vi "SwerveDrive2.0.vi"(6 "Right Trigger":dbl, 8 "RCW":dbl(slide) scale=-1.0..1.0, 9 "STR":dbl(slide) scale=-1.0..1.0, 10 "FWD":dbl(slide) scale=-1.0..1.0, 11 "Gyro":dbl) -> ()   [LabVIEW 2020]
uses:
  <vilib>/Rock Robotics/WPI/ThirdParty/ADI/ADIS16470/Typedef/ADIS16470 Data.ctl
  <vilib>/addons/control/pid/pid.llb/PID (DBL).vi
  <vilib>/addons/control/pid/NI_PID_pid.lvlib
panel:
  in  "Do X Pattern":bool
  out "Goal 4":dbl
  out "Goal 3":dbl
  out "Goal 2":dbl
  out "Goal 1":dbl
  in  "W4 PID":T1={"proportional gain (Kc)"=0.5, "integral time (Ti, min)"=0.0, "derivative time (Td, min)"=0.0}
  in  "W1 PID":T1={"proportional gain (Kc)"=0.5, "integral time (Ti, min)"=0.0, "derivative time (Td, min)"=0.0}
  in  "W2 PID":T1={"proportional gain (Kc)"=0.5, "integral time (Ti, min)"=0.0, "derivative time (Td, min)"=0.0}
  in  "W3 PID":T1={"proportional gain (Kc)"=0.5, "integral time (Ti, min)"=0.0, "derivative time (Td, min)"=0.0}
  out "ADIS16470 Value":T2
  out "W2 Encoder":dbl
  out "W1 Encoder":dbl
  out "WA 4":dbl
  out "WA 3":dbl
  out "WA 2":dbl
  out "WA 1":dbl
  out "WS 4":dbl
  out "WS 3":dbl
  out "WS 2":dbl
  out "WS 1":dbl
  out "W4 Encoder":dbl
  out "W3 Encoder":dbl
  # "0.5\n0\n0\nfor all"
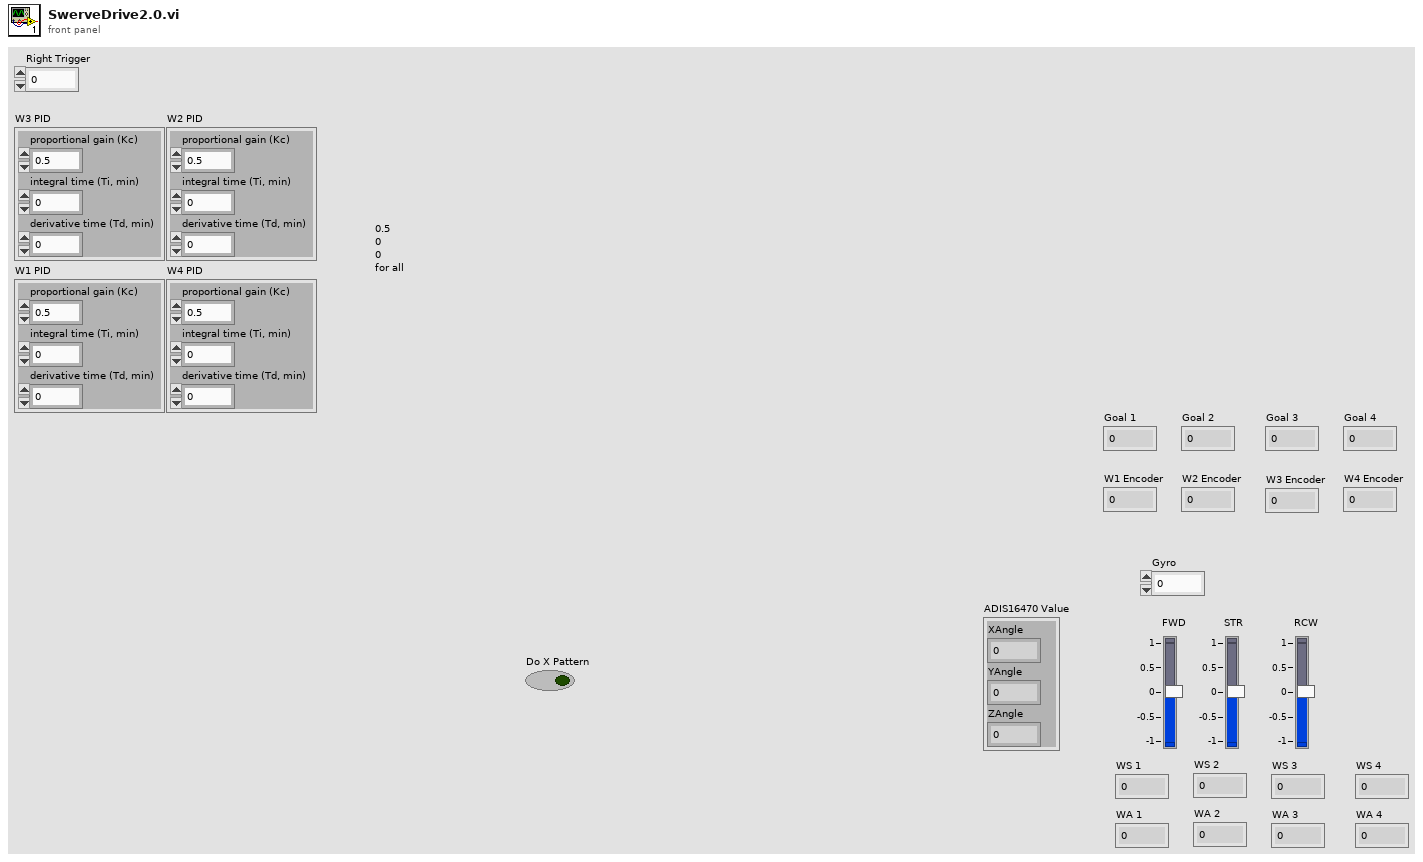
[diagram p1: front panel]
types:
  T1 = cluster{"proportional gain (Kc)":dbl, "integral time (Ti, min)":dbl, "derivative time (Td, min)":dbl}
  T2 = typedef "ADIS16470 Data.ctl" = cluster{"XAngle":dbl, "YAngle":dbl, "ZAngle":dbl}
  T3 = typedef "WPI_JoystickDevRef.ctl" = cluster{"Device":T4}
  T4 = typedef "WPI_JoystickDeviceEnum.ctl" = enum16{"USB 0", "USB 1", "USB 2", "USB 3", "USB 4", "USB 5"}
  T5 = typedef "ADIS16470 Device Reference.ctl" = cluster{"DevStatus":errorcluster, "Hardware Config":T6, "Calibration Complete":refnum<notifier>, "Status Reference":refnum<data-value>, "Data Reference":refnum<data-value>, "Sychronous Process VI":T10, "Cmd FIFO":refnum<k33>, "Source":T11, "Data FIFO":refnum<k33>, "Calibration Time (ms)":u32, "Data Reference":refnum<data-value>}
  T6 = typedef "ADIS16470 Hardware Configuration.ctl" = cluster{"SPI Clock Rate (Hz)":dbl, "IMU SPI Mode (3)":T7, "IMU Reset Pin":T8, "IMU SPI Bus":T9, "IMU Data Ready Pin":T8, "Stall Config":cluster{"Pow2BytesPerRead":u8, "StallTicks":u16, "CsToSclkTicks":u8}}
  T7 = typedef "WPI_SPIMode.ctl" = enum16{"Mode 0 (Clk Idle Low,Sample on Leading)", "Mode 1 (Clk Idle Low,Sample on Trailing)", "Mode 2 (Clk Idle High,Sample on Leading)", "Mode 3 (Clk Idle High,Sample on Trailing)"}
  T8 = typedef "FPGA_DIOChannel.ctl" = enum8{"DIO 0", "DIO 1", "DIO 2", "DIO 3", "DIO 4", "DIO 5", "DIO 6", "DIO 7", "DIO 8", "DIO 9", "DIO MXP 0", "DIO MXP 1", "DIO MXP 2", "DIO MXP 3", "DIO MXP 4", "DIO MXP 5", "DIO MXP 6", "DIO MXP 7", "DIO MXP 8", "DIO MXP 9", "DIO MXP 10", "DIO MXP 11", "DIO MXP 12", "DIO MXP 13", "DIO MXP 14", "DIO MXP 15", "SPI Port CS1", "SPI Port CS2", "SPI Port CS3", "SPI Port MISO", "SPI Port MOSI", "Invalid"}
  T9 = typedef "spi_bus.ctl" = enum16{"SPI On-Board, CS0", "SPI On-Board, CS1", "SPI On-Board, CS2", "SPI On-Board, CS3", "SPI MXP", "Invalid"}
  T10 = typedef "ADIS16470 Process.ctl" = refnum<vi>
  T11 = typedef "FPGA_CounterEncoderSourceConvertionLVSourceType.ctl" = cluster{"DevStatus":errorcluster, "AnalogTriggerMode?":bool, "DigitalMode":cluster{"DIO Channel":T12}, "AnalogTriggerMode":cluster{"AnalogTriggerIndex":T13, "OutputType":T14}}
  T12 = typedef "FPGA_DIODigitalSourceChannel.ctl" = enum8{"DIO 0", "DIO 1", "DIO 2", "DIO 3", "DIO 4", "DIO 5", "DIO 6", "DIO 7", "DIO 8", "DIO 9", "DIO MXP 0", "DIO MXP 1", "DIO MXP 2", "DIO MXP 3", "DIO MXP 4", "DIO MXP 5", "DIO MXP 6", "DIO MXP 7", "DIO MXP 8", "DIO MXP 9", "DIO MXP 10", "DIO MXP 11", "DIO MXP 12", "DIO MXP 13", "DIO MXP 14", "DIO MXP 15", "SPI Port CS1", "SPI Port CS2", "SPI Port CS3", "SPI Port MISO", "SPI Port MOSI", "Disabled"}
  T13 = typedef "FPGA_AnalogTriggerIndex.ctl" = enum8{"Trig 0", "Trig 1", "Trig 2", "Trig 3", "Trig 4", "Trig 5", "Trig 6", "Trig 7", "Invalid"}
  T14 = typedef "FPGA_AnalogTriggerOutType.ctl" = enum16{"InWindow", "TriggerState", "Rising", "Falling"}
  T15 = typedef "WPI_MotorControlDeviceRef.ctl" = cluster{"DeviceStatus":errorcluster, "Type":T16, "PWM":cluster{"PWM Channel":T17, "DeadBand":T18}, "CAN":cluster{"Device Number":u8, "SetOutput VI Ref":variant, "GetOutput VI Ref":variant, "Enable VI Ref":variant, "Disable VI Ref":variant, "Data":variant}, "Invert":bool, "DIO PWM":cluster{"PWM \"Enable\" Channel":T17, "DIOChannel":T8, "PWM Rate":dbl}}
  T16 = typedef "WPI_MotorControlType.ctl" = enum16{"PWM", "CAN", "DIO PWM"}
  T17 = typedef "FPGA_DIOPWMChannel.ctl" = enum8{"PWM 0", "PWM 1", "PWM 2", "PWM 3", "PWM 4", "PWM 5", "PWM 6", "PWM 7", "PWM 8", "PWM 9", "PWM MXP 0", "PWM MXP 1", "PWM MXP 2", "PWM MXP 3", "PWM MXP 4", "PWM MXP 5", "PWM MXP 6", "PWM MXP 7", "PWM MXP 8", "PWM MXP 9", "Invalid"}
  T18 = typedef "WPI_PWMDeadband.ctl" = cluster{"Name":string, "maxPositivePwm":i32, "minPositivePwm":i32, "centerPwm":i32, "maxNegativePwm":i32, "minNegativePwm":i32, "angularRange":u16}
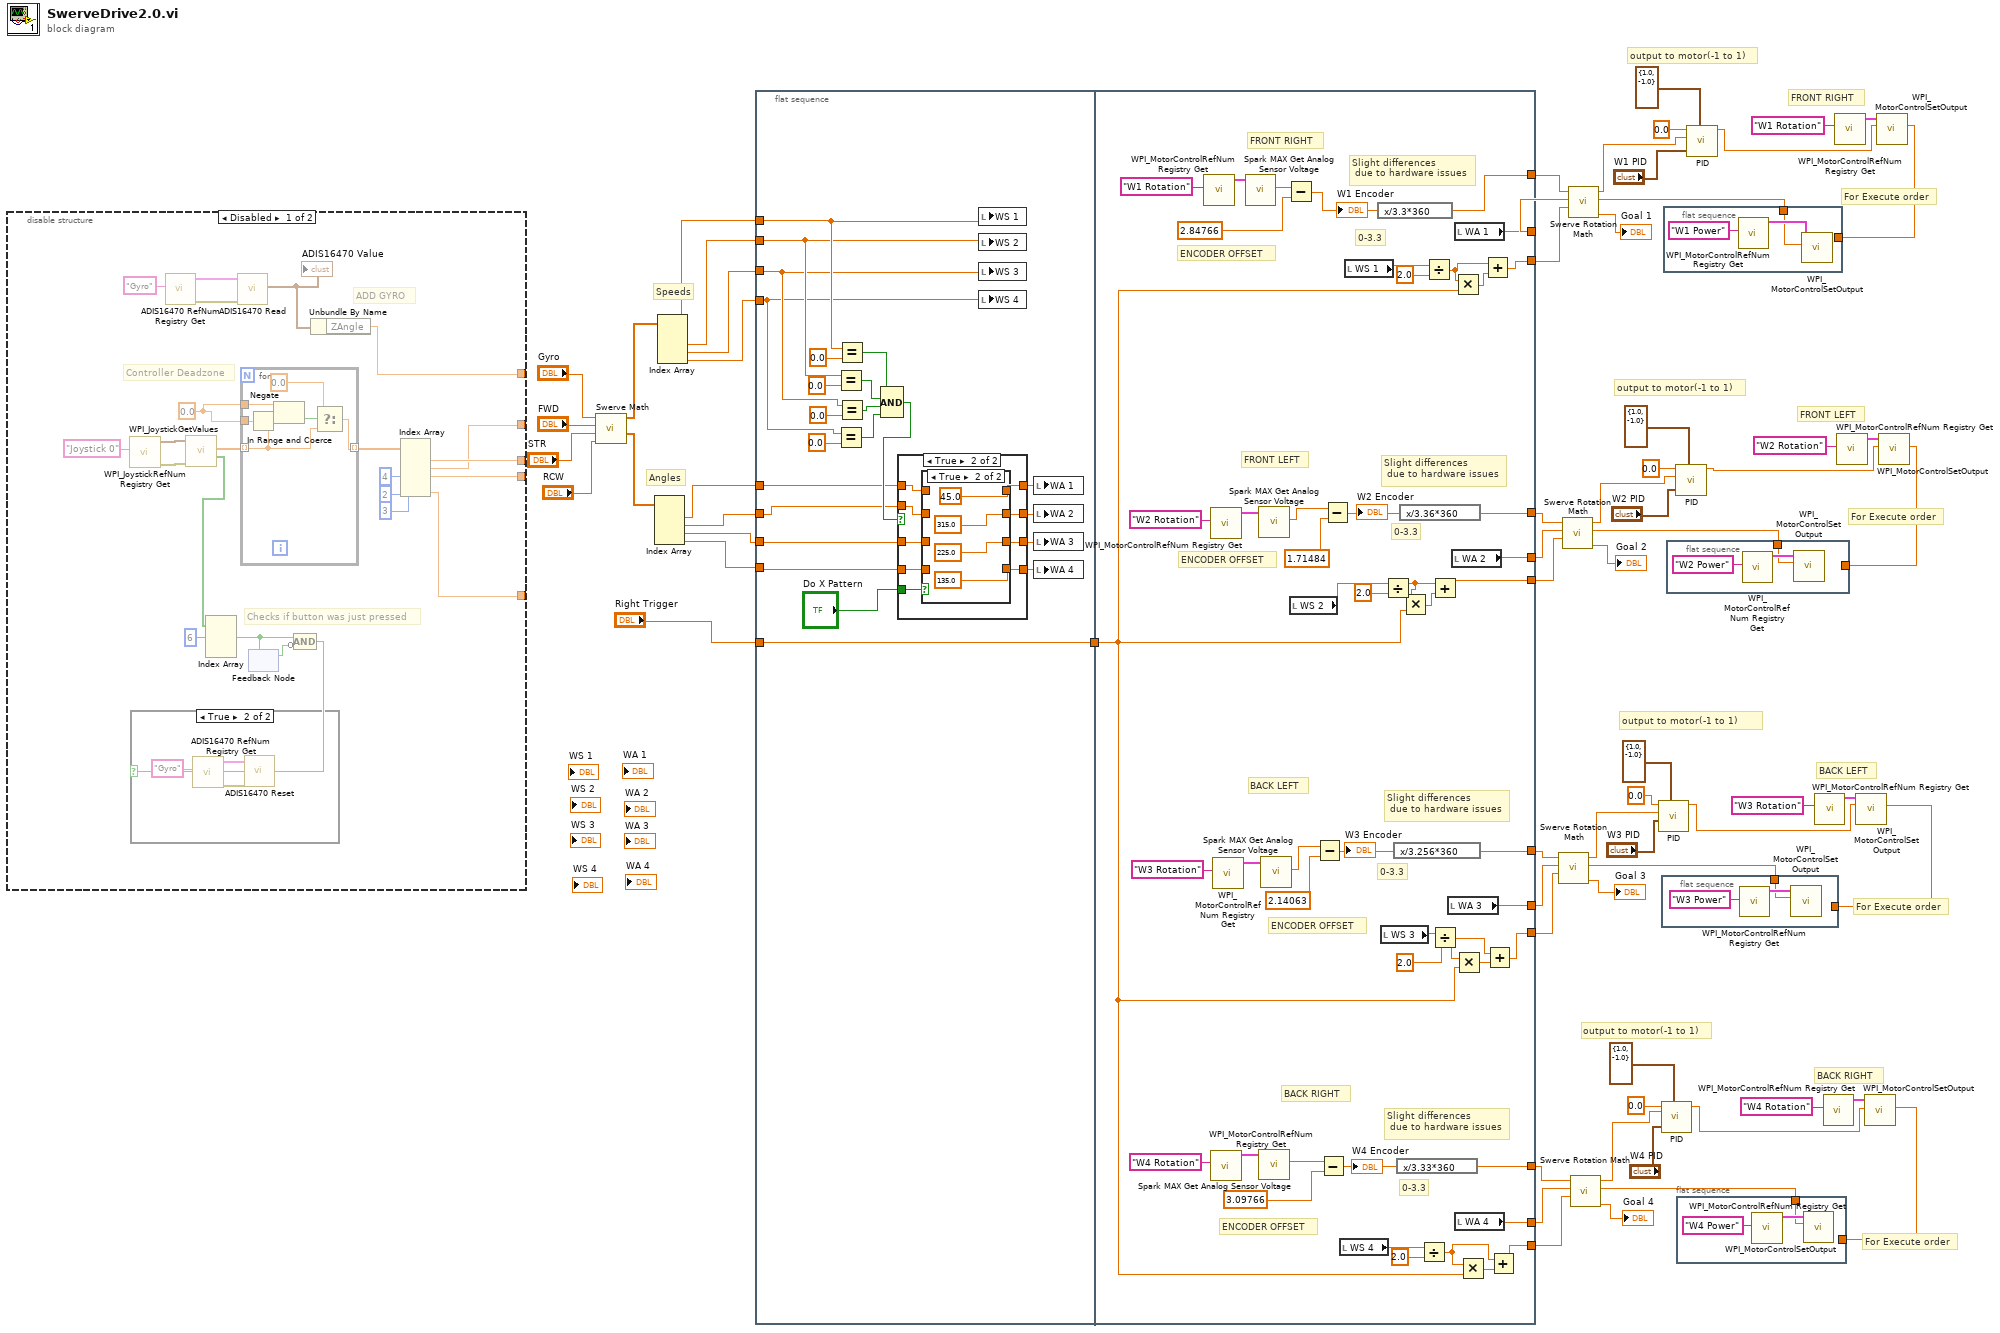
[diagram p0: block diagram]
diagram:
  # "output to motor(-1 to 1)"
  # "BACK RIGHT"
  # "BACK LEFT"
  # "FRONT LEFT"
  # "FRONT RIGHT"
  # "output to motor(-1 to 1)"
  # "output to motor(-1 to 1)"
  # "output to motor(-1 to 1)"
  # "For Execute order"
  # "For Execute order"
  # "For Execute order"
  # "For Execute order"
  # "Angles"
  # "Speeds"
  n1 = disable-structure shown="Disabled" {
    disable-tunnel: [w88 _] -> _
    disable-tunnel: [w87 _] -> _
    disable-tunnel: [w86 _] -> _
    disable-tunnel: [w75 _] -> _
    disable-tunnel: [w72 _] -> _
    frame Disabled {
      w81 = 0.0 ("upper limit")
      # "Checks if button was just pressed"
      # "Controller Deadzone"
      # "ADD GYRO"
      n2 = call <vilib>:"WPI_JoystickRefNum Registry Get.vi"("refnum name"="Joystick 0") -> ("error out"=w91:errorcluster, "JoystickDevRef"=w90:T3)  [unwired: 9 in]
      n3 = call <vilib>:"ADIS16470 RefNum Registry Get.vi"("refnum name"="Gyro") -> ("error out"=w71:errorcluster, "ADIS16470DevRef out"=w69:T5)  [unwired: 9 in]
      n4 = call <vilib>:"WPI_JoystickGetValues.vi"("error in (no error)"=w91, "JoystickDevRef"=w90) -> ("Buttons"=w80:bool[], "Axes"=w83:dbl[])  [unwired: 5 in, 3 out]
      n5 = Index Array(array=w80, index #1=6 ("index")) -> (element #1=w78:bool)  [unwired: 2 in, 2 out]
      n6 = call <vilib>:"ADIS16470 Read.vi"("error in (no error)"=w71, "ADIS16470DevRef"=w69) -> ("ADIS16470 Value"=w84:T2)  [unwired: 6 in, 3 out]
      "ADIS16470 Value" <- w84
      n7 = for {
        tunnel: w83 -> [w96] mode=indexing
        tunnel: [w95] -> w82 mode=indexing
        tunnel: w81 -> [w101]
        tunnel: w81 -> [w100]
        n8 = Negate(x=w100) -> (-x=w99:dbl)
        n9 = In Range and Coerce(upper limit=w101, x=w96, lower limit=w99) -> (In Range?=w98:bool)  [unwired: 1 out]
        n10 = Select(t=0.0, s=w98, f=w96) -> (s? t:f=w95:dbl)
      }
      n11 = feedback #1() -> (w77:bool)  [unwired: 1 in]
      n12 = feedback-in #1(w78) -> ()
      n13 = Compound Arithmetic op=AND(w78, invert w77) -> (w76:bool)
      n14 = case shown="True" w76 {
        frame False {
        }
        frame True {
          n15 = call <vilib>:"ADIS16470 RefNum Registry Get.vi"("refnum name"="Gyro") -> ("error out"=w93:errorcluster, "ADIS16470DevRef out"=w92:T5)  [unwired: 9 in]
          n16 = call <vilib>:"ADIS16470 Reset.vi"("error in (no error)"=w93, "ADIS16470DevRef"=w92) -> ()  [unwired: 8 in, 2 out]
        }
      }
      n17 = Unbundle By Name(w84) -> ("ZAngle"=w75:dbl)
      n18 = Index Array(array=w82, index #3=4 ("index"), index #4=2 ("index"), index #5=3 ("index")) -> (element #1=w88:dbl, element #2=w86:dbl, element #3=w87:dbl, element #5=w72:dbl)  [unwired: 2 in, 1 out]
    }
    frame Enabled {
    }
  }
  n19 = call "Swerve Math.vi"("Gyro"="Gyro", "FWD"="FWD", "STR"="STR", "RCW"="RCW") -> ("Wheel Speeds"=w68:dbl[], "Wheel Angles"=w67:dbl[])  [unwired: 5 in]
  n20 = Index Array(array=w67) -> (element #1=w51:dbl, element #2=w52:dbl, element #3=w53:dbl, element #4=w54:dbl)  [unwired: 4 in]
  n21 = Index Array(array=w68) -> (element #1=w49:dbl, element #2=w3:dbl, element #3=w4:dbl, element #4=w50:dbl)  [unwired: 4 in]
  n22 = flat-sequence {
    tunnel: w54 -> [w103]
    tunnel: w53 -> [w106]
    tunnel: w52 -> [w108]
    tunnel: w51 -> [w110]
    tunnel: w50 -> [w112]
    tunnel: w4 -> [w113]
    tunnel: w49 -> [w115]
    tunnel: w3 -> [w114]
    tunnel: "Right Trigger" -> [w124]
    tunnel: [w124] -> w2
    tunnel: [w194] -> w47
    tunnel: [w193] -> w41
    tunnel: [w192] -> w35
    tunnel: [w191] -> w30
    tunnel: [w190] -> w36
    tunnel: [w189] -> w28
    tunnel: [w172] -> w42
    tunnel: [w171] -> w48
    tunnel: [w154] -> w46
    tunnel: [w158] -> w40
    tunnel: [w150] -> w34
    tunnel: [w148] -> w29
    tunnel: w2 -> [w146]
    frame #0 {
      n23 = Equal?(x=w114, y=0.0) -> (x = y?=w120:bool)
      n24 = Equal?(x=w112, y=0.0) -> (x = y?=w116:bool)
      n25 = Equal?(x=w115, y=0.0) -> (x = y?=w123:bool)
      n26 = Equal?(x=w113, y=0.0) -> (x = y?=w117:bool)
      n27 = Compound Arithmetic op=AND(w123, w120, w117, w116) -> (w111:bool)
      n28 = case shown="True" w111 {
        tunnel: w110 -> [w128 w132]
        tunnel: [w128 w137] -> w109
        tunnel: w108 -> [w127 w131]
        tunnel: [w127 w136] -> w107
        tunnel: w106 -> [w126 w130]
        tunnel: [w126 w135] -> w105
        tunnel: w103 -> [w125 w129]
        tunnel: [w125 w134] -> w104
        tunnel: "Do X Pattern" -> [_ w133]
        frame False {
        }
        frame True {
          n29 = case shown="True" w133 {
            tunnel: [w141 45.0] -> w137
            tunnel: [w140 315.0] -> w136
            tunnel: [w139 225.0] -> w135
            tunnel: [w138 135.0] -> w134
            tunnel: w132 -> [w141 _]
            tunnel: w131 -> [w140 _]
            tunnel: w130 -> [w139 _]
            tunnel: w129 -> [w138 _]
            frame False {
            }
            frame True {
            }
          }
        }
      }
      n30 = local write "WS 1"(w115) -> ()
      n31 = local write "WS 2"(w114) -> ()
      n32 = local write "WS 3"(w113) -> ()
      n33 = local write "WS 4"(w112) -> ()
      n34 = local write "WA 1"(w109) -> ()
      n35 = local write "WA 2"(w107) -> ()
      n36 = local write "WA 3"(w105) -> ()
      n37 = local write "WA 4"(w104) -> ()
    }
    frame #1 {
      # "Slight differences\n due to hardware issues"
      # "Slight differences\n due to hardware issues"
      # "Slight differences\n due to hardware issues"
      # "Slight differences\n due to hardware issues"
      # "BACK RIGHT"
      # "BACK LEFT"
      # "FRONT LEFT"
      # "FRONT RIGHT"
      # "ENCODER OFFSET"
      # "ENCODER OFFSET"
      # "ENCODER OFFSET"
      # "ENCODER OFFSET"
      # "0-3.3"
      # "0-3.3"
      # "0-3.3"
      # "0-3.3"
      n38 = call <vilib>:"WPI_MotorControlRefNum Registry Get.vi"("refnum name"="W1 Rotation") -> ("MotorControlDevRef"=w188:T15)  [unwired: 9 in, 1 out]
      n39 = call <vilib>:"WPI_MotorControlRefNum Registry Get.vi"("refnum name"="W2 Rotation") -> ("MotorControlDevRef"=w173:T15)  [unwired: 9 in, 1 out]
      n40 = call <vilib>:"WPI_MotorControlRefNum Registry Get.vi"("refnum name"="W4 Rotation") -> ("MotorControlDevRef"=w183:T15)  [unwired: 9 in, 1 out]
      n41 = call <vilib>:"WPI_MotorControlRefNum Registry Get.vi"("refnum name"="W3 Rotation") -> ("MotorControlDevRef"=w185:T15)  [unwired: 9 in, 1 out]
      n42 = call <vilib>:"Spark MAX Get Analog Sensor Voltage.vi"("MotorControlDevRef in"=w188) -> ("Analog Sensor Voltage"=w180:dbl)  [unwired: 7 in, 3 out]
      n43 = call <vilib>:"Spark MAX Get Analog Sensor Voltage.vi"("MotorControlDevRef in"=w173) -> ("Analog Sensor Voltage"=w178:dbl)  [unwired: 7 in, 3 out]
      n44 = call <vilib>:"Spark MAX Get Analog Sensor Voltage.vi"("MotorControlDevRef in"=w183) -> ("Analog Sensor Voltage"=w179:dbl)  [unwired: 7 in, 3 out]
      n45 = call <vilib>:"Spark MAX Get Analog Sensor Voltage.vi"("MotorControlDevRef in"=w185) -> ("Analog Sensor Voltage"=w181:dbl)  [unwired: 7 in, 3 out]
      n46 = Subtract(x=w180, y=2.84766) -> (x-y=w166:dbl)
      "W1 Encoder" <- w166
      n47 = local read "WS 2"() -> (w176:dbl)
      n48 = Subtract(x=w181, y=2.14063) -> (x-y=w164:dbl)
      "W3 Encoder" <- w164
      n49 = Subtract(x=w179, y=3.09766 ("x")) -> (x-y=w163:dbl)
      "W4 Encoder" <- w163
      n50 = Subtract(x=w178, y=1.71484) -> (x-y=w165:dbl)
      "W2 Encoder" <- w165
      n51 = local read "WS 4"() -> (w174:dbl)
      n52 = local read "WS 1"() -> (w177:dbl)
      n53 = expression code="x/3.3*360"(w166) -> (w171:dbl)
      n54 = local read "WS 3"() -> (w175:dbl)
      n55 = Divide(x=w176, y=2.0) -> (x/y=w156:dbl)
      n56 = expression code="x/3.256*360"(w164) -> (w190:dbl)
      n57 = expression code="x/3.33*360"(w163) -> (w189:dbl)
      n58 = expression code="x/3.36*360"(w165) -> (w172:dbl)
      n59 = Multiply(x=w156, y=w146) -> (x*y=w157:dbl)
      n60 = Divide(x=w174, y=2.0) -> (x/y=w147:dbl)
      n61 = Divide(x=w177, y=2.0) -> (x/y=w153:dbl)
      n62 = Add(x=w156, y=w157) -> (x+y=w158:dbl)
      n63 = Divide(x=w175, y=2.0) -> (x/y=w151:dbl)
      n64 = local read "WA 3"() -> (w192:dbl)
      n65 = local read "WA 2"() -> (w193:dbl)
      n66 = Multiply(x=w153, y=w146) -> (x*y=w155:dbl)
      n67 = Multiply(x=w151, y=w146) -> (x*y=w152:dbl)
      n68 = local read "WA 1"() -> (w194:dbl)
      n69 = local read "WA 4"() -> (w191:dbl)
      n70 = Multiply(x=w147, y=w146) -> (x*y=w149:dbl)
      n71 = Add(x=w153, y=w155) -> (x+y=w154:dbl)
      n72 = Add(x=w151, y=w152) -> (x+y=w150:dbl)
      n73 = Add(x=w147, y=w149) -> (x+y=w148:dbl)
    }
  }
  n74 = call "Swerve Rotation Math.vi"("Wheel Speed"=w34, "Wheel Angle"=w35, "Encoder"=w36) -> ("Goal"=→"Goal 3":dbl, "Wheel Speed"=w32:dbl, "Difference"=w33:dbl)  [unwired: 6 in]
  n75 = call "Swerve Rotation Math.vi"("Wheel Speed"=w40, "Wheel Angle"=w41, "Encoder"=w42) -> ("Goal"=→"Goal 2":dbl, "Wheel Speed"=w38:dbl, "Difference"=w39:dbl)  [unwired: 6 in]
  n76 = call "Swerve Rotation Math.vi"("Wheel Speed"=w46, "Wheel Angle"=w47, "Encoder"=w48) -> ("Goal"=→"Goal 1":dbl, "Wheel Speed"=w44:dbl, "Difference"=w43:dbl)  [unwired: 6 in]
  n77 = call "Swerve Rotation Math.vi"("Wheel Speed"=w29, "Wheel Angle"=w30, "Encoder"=w28) -> ("Goal"=→"Goal 4":dbl, "Wheel Speed"=w9:dbl, "Difference"=w26:dbl)  [unwired: 6 in]
  n78 = call-poly <vilib>:"PID.vi"("output range"=cluster{"output high":dbl, "output low":dbl} {"output high"=1.0, "output low"=-1.0}, "PID gains"="W3 PID", "process variable"=w33, "setpoint"=0.0) -> ("output"=w16:dbl)  [unwired: 6 in, 1 out]
  n79 = flat-sequence {
    tunnel: w14 -> [_]
    tunnel: w32 -> [w195]
    frame #0 {
      n80 = call <vilib>:"WPI_MotorControlRefNum Registry Get.vi"("refnum name"="W3 Power") -> ("MotorControlDevRef"=w196:T15)  [unwired: 9 in, 1 out]
      n81 = call <vilib>:"WPI_MotorControlSetOutput.vi"("Output"=w195, "MotorControlDevRef"=w196) -> ()  [unwired: 7 in, 3 out]
    }
  }
  n82 = call-poly <vilib>:"PID.vi"("output range"=cluster{"output high":dbl, "output low":dbl} {"output high"=1.0, "output low"=-1.0}, "PID gains"="W4 PID", "process variable"=w26, "setpoint"=0.0) -> ("output"=w12:dbl)  [unwired: 6 in, 1 out]
  n83 = flat-sequence {
    tunnel: w22 -> [_]
    tunnel: w44 -> [w198]
    frame #0 {
      n84 = call <vilib>:"WPI_MotorControlRefNum Registry Get.vi"("refnum name"="W1 Power") -> ("MotorControlDevRef"=w199:T15)  [unwired: 9 in, 1 out]
      n85 = call <vilib>:"WPI_MotorControlSetOutput.vi"("Output"=w198, "MotorControlDevRef"=w199) -> ()  [unwired: 7 in, 3 out]
    }
  }
  n86 = flat-sequence {
    tunnel: w18 -> [_]
    tunnel: w38 -> [w201]
    frame #0 {
      n87 = call <vilib>:"WPI_MotorControlRefNum Registry Get.vi"("refnum name"="W2 Power") -> ("MotorControlDevRef"=w202:T15)  [unwired: 9 in, 1 out]
      n88 = call <vilib>:"WPI_MotorControlSetOutput.vi"("Output"=w201, "MotorControlDevRef"=w202) -> ()  [unwired: 7 in, 3 out]
    }
  }
  n89 = call-poly <vilib>:"PID.vi"("output range"=cluster{"output high":dbl, "output low":dbl} {"output high"=1.0, "output low"=-1.0}, "PID gains"="W2 PID", "process variable"=w39, "setpoint"=0.0) -> ("output"=w20:dbl)  [unwired: 6 in, 1 out]
  n90 = flat-sequence {
    tunnel: w10 -> [_]
    tunnel: w9 -> [w204]
    frame #0 {
      n91 = call <vilib>:"WPI_MotorControlRefNum Registry Get.vi"("refnum name"="W4 Power") -> ("MotorControlDevRef"=w205:T15)  [unwired: 9 in, 1 out]
      n92 = call <vilib>:"WPI_MotorControlSetOutput.vi"("Output"=w204, "MotorControlDevRef"=w205) -> ()  [unwired: 7 in, 3 out]
    }
  }
  n93 = call-poly <vilib>:"PID.vi"("output range"=cluster{"output high":dbl, "output low":dbl} {"output high"=1.0, "output low"=-1.0}, "PID gains"="W1 PID", "process variable"=w43, "setpoint"=0.0) -> ("output"=w24:dbl)  [unwired: 6 in, 1 out]
  n94 = call <vilib>:"WPI_MotorControlRefNum Registry Get.vi"("refnum name"="W3 Rotation") -> ("MotorControlDevRef"=w17:T15)  [unwired: 9 in, 1 out]
  n95 = call <vilib>:"WPI_MotorControlRefNum Registry Get.vi"("refnum name"="W4 Rotation") -> ("MotorControlDevRef"=w13:T15)  [unwired: 9 in, 1 out]
  n96 = call <vilib>:"WPI_MotorControlRefNum Registry Get.vi"("refnum name"="W1 Rotation") -> ("MotorControlDevRef"=w25:T15)  [unwired: 9 in, 1 out]
  n97 = call <vilib>:"WPI_MotorControlRefNum Registry Get.vi"("refnum name"="W2 Rotation") -> ("MotorControlDevRef"=w21:T15)  [unwired: 9 in, 1 out]
  n98 = call <vilib>:"WPI_MotorControlSetOutput.vi"("Output"=w16, "MotorControlDevRef"=w17) -> ("Motor Output"=w14:dbl)  [unwired: 7 in, 2 out]
  n99 = call <vilib>:"WPI_MotorControlSetOutput.vi"("Output"=w12, "MotorControlDevRef"=w13) -> ("Motor Output"=w10:dbl)  [unwired: 7 in, 2 out]
  n100 = call <vilib>:"WPI_MotorControlSetOutput.vi"("Output"=w24, "MotorControlDevRef"=w25) -> ("Motor Output"=w22:dbl)  [unwired: 7 in, 2 out]
  n101 = call <vilib>:"WPI_MotorControlSetOutput.vi"("Output"=w20, "MotorControlDevRef"=w21) -> ("Motor Output"=w18:dbl)  [unwired: 7 in, 2 out]
